vi "Table_MoveNumericToCell.vi"(6 "Data":string[][](array[string]), 8 "error in (no error)":errorcluster, 9 "Numeric":refnum<vi>, 10 "Cell Position":T1, 11 "Listbox":refnum<vi>) -> (0 "error out":errorcluster)   [LabVIEW 2012, in "TableSupportLib.lvlib"]
uses:
  TableSupportLib.lvlib
  <vilib>/Utility/miscctls.llb/LVRowAndColumnTypeDef.ctl
  Table_Globals.vi
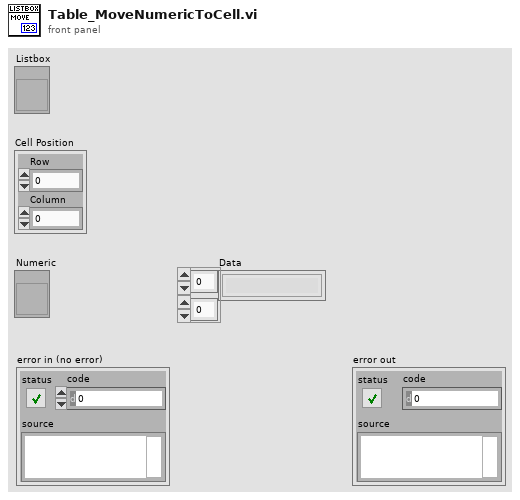
[diagram p1: front panel]
types:
  T1 = typedef "LVRowAndColumnTypeDef.ctl" = cluster{"Row":i32, "Column":i32}
  T2 = typedef "LVBoundsTypeDef.ctl" = cluster{"Width":u32, "Height":u32}
  T3 = typedef "LVPositionTypeDef.ctl" = cluster{"Left":i32, "Top":i32}
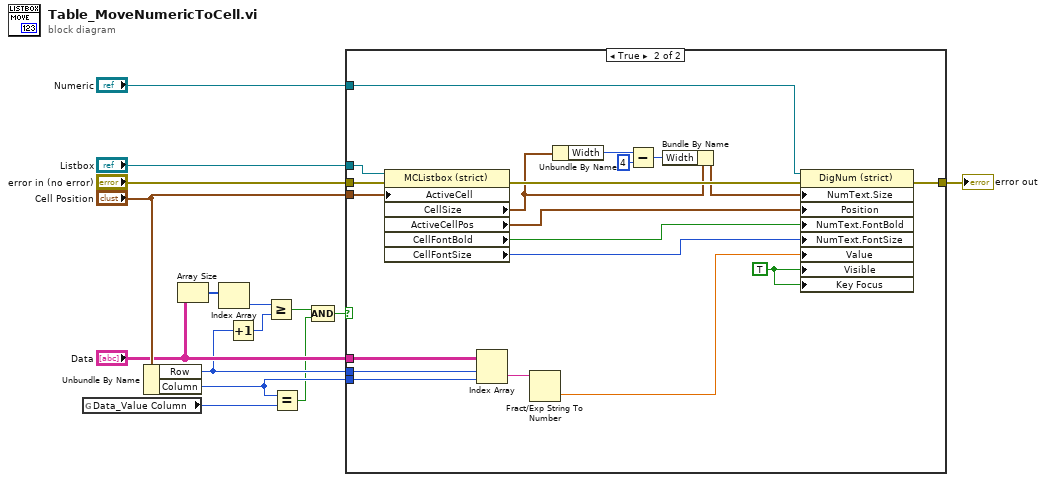
[diagram p0: block diagram]
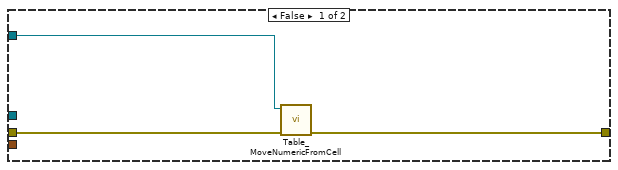
[diagram p2: hidden frame]
diagram:
  n1 = global read "Table_Globals.vi" "Data_Value Column"() -> (w5:i32)
  n2 = Unbundle By Name("Cell Position") -> ("Row"=w6:i32, "Column"=w4:i32)
  n3 = Array Size(array="Data") -> (size(s)=w9:i32[])
  n4 = Index Array(array=w9) -> (element=w8:i32)  [unwired: 1 in]
  n5 = Increment(x=w6) -> (x+1=w1:i32)
  n6 = Greater Or Equal?(x=w8, y=w1) -> (x >= y?=w7:bool)
  n7 = Equal?(x=w4, y=w5) -> (x = y?=w2:bool)
  n8 = Compound Arithmetic op=AND(w7, w2) -> (w3:bool)
  n9 = case shown="True" w3 {
    tunnel: "Listbox" -> [_ w38]
    tunnel: "Numeric" -> [w18 w37]
    tunnel: "error in (no error)" -> [w17 w35]
    tunnel: [w16 w33] -> w12
    tunnel: "Cell Position" -> [_ w31]
    tunnel: w6 -> [_ w30]
    tunnel: w4 -> [_ w29]
    tunnel: "Data" -> [_ w19]
    frame False {
      n10 = call "Table_MoveNumericFromCell.vi"("error in (no error)"=w17, "Digital in"=w18) -> ("error out"=w16:errorcluster)  [unwired: 9 in]
    }
    frame True {
      w26 = TRUE ("Visible")
      n11 = property class="MCListbox (strict)"(reference=w38, error in=w35, "ActiveCell"=w31) -> (error out=w34:errorcluster, "CellSize"=w22:T2, "ActiveCellPos"=w25:T3, "CellFontBold"=w36:bool, "CellFontSize"=w32:u32)  [unwired: 1 out]
      n12 = Index Array(array=w19, index (row)=w30, index (col)=w29) -> (element=w28:string)
      n13 = Fract/Exp String To Number(string=w28) -> (number=w27:dbl)  [unwired: 3 in, 1 out]
      n14 = Unbundle By Name(w22) -> ("Width"=w24:u32)
      n15 = Subtract(x=w24, y=u32 4) -> (x-y=w20:u32)
      n16 = Bundle By Name(cluster=w22, "Width"=w20) -> (w21:T2)
      n17 = property class="DigNum (strict)"(reference=w37, error in=w34, "NumText.Size"=w21, "Position"=w25, "NumText.FontBold"=w36, "NumText.FontSize"=w32, "Value"=w27, "Visible"=w26, "Key Focus"=w26) -> (error out=w33:errorcluster)  [unwired: 1 out]
    }
  }
  "error out" <- w12
